vi "Conjunto_2.vi"() -> ()   [LabVIEW 2016]
panel:
  out "subarray":bool[](array[boolean])
  in  "Array":bool[](array[boolean])
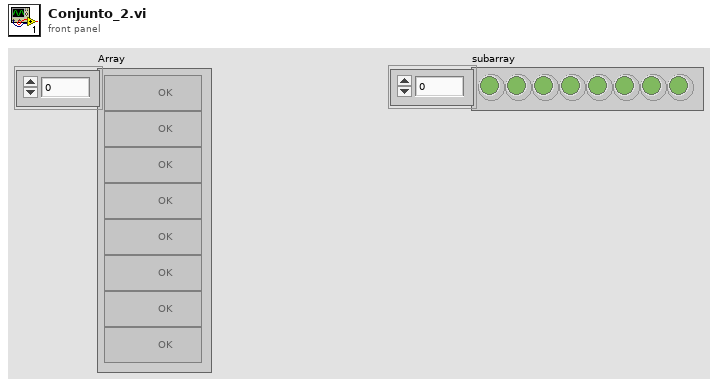
[diagram p1: front panel]
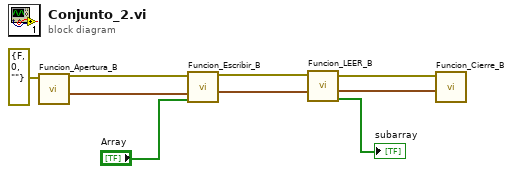
[diagram p0: block diagram]
diagram:
  n1 = call <userlib>:"Funcion_Apertura_B.vi"("error in (no error)"=errorcluster {"status"=FALSE, "code"=0, "source"=""}) -> ("PIPES"=w7:cluster{"PIPE_IN":i32, "PIPE_OUT":i32}, "error out"=w9:errorcluster)  [unwired: 8 in, 1 out]
  n2 = call <userlib>:"Funcion_Escribir_B.vi"("Array"="Array", "PIPES ENTRADA"=w7, "error in (no error)"=w9) -> ("PIPES SALIDA"=w6:cluster{"PIPE_IN":i32, "PIPE_OUT":i32}, "error out"=w3:errorcluster)  [unwired: 7 in]
  n3 = call <userlib>:"Funcion_LEER_B.vi"("PIPES ENTRADA"=w6, "error in (no error)"=w3) -> ("subarray"=→"subarray":bool[], "PIPES SALIDA"=w5:cluster{"PIPE_IN":i32, "PIPE_OUT":i32}, "error out"=w4:errorcluster)  [unwired: 7 in]
  n4 = call <userlib>:"Funcion_Cierre_B.vi"("PIPES"=w5, "error in (no error)"=w4) -> ()  [unwired: 8 in, 2 out]
